vi "Configure Chan Input.vi"(6 "Gate Mode (0:Disabled)":T1(ring), 7 "Channel (1:Chan A)":i32(ring)=1 items=["Channel A"=1, "Channel B"=2, "Channel C"=3, "Channel D"=4, "Channel E"=5, "Channel F"=6, "Channel G"=7, "Channel H"=8], 8 "error in (no error)":errorcluster, 9 "Gate Logic (0:Disabled)":enum16{"Disabled", "Low", "High"}(ring), 10 "Sync Source (0:To)":i32(ring) items=["System (To)", "Channel A", "Channel B", "Channel C", "Channel D", "Channel E", "Channel F", "Channel G", "Channel H"], 11 "VISA resource name":refnum<visa-resource-name>) -> (0 "error out":errorcluster, 3 "VISA resource name out":refnum<visa-resource-name>)   [LabVIEW 2012, in "Berkeley Nucleonics 500 Series.lvlib"]
doc: "This VI is used to configure the gate mode for a channel."
uses:
  Berkeley Nucleonics 500 Series.lvlib
panel:
  # "The \"Gate Mode\" input is currently only utilized by 9520/9530 instruments.  When controlling a 9520/9530, the \"Gate Logic\" disabled setting is ignored."
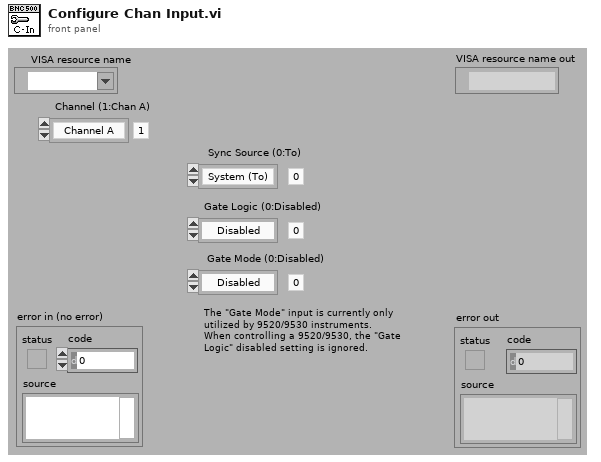
[diagram p1: front panel]
types:
  T1 = enum16{"Disabled", "Pulse Inhibit", "Output Inhibit"}
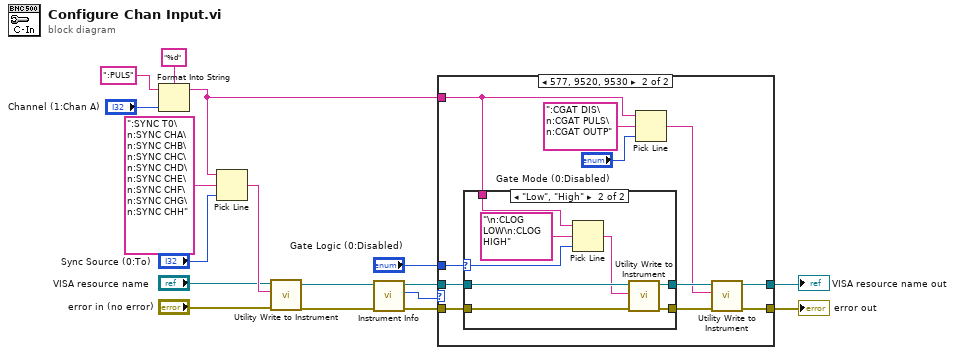
[diagram p0: block diagram]
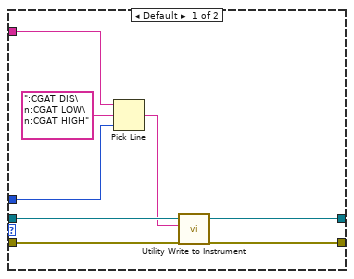
[diagram p2: hidden frame]
diagram:
  n1 = Format Into String(format string="%d", initial string=":PULS", "Channel (1:Chan A)") -> (resulting string=w5:string)  [unwired: 1 in, 1 out]
  n2 = Pick Line(string ("")=w5, multi-line string=":SYNC T0\n:SYNC CHA\n:SYNC CHB\n:SYNC CHC\n:SYNC CHD\n:SYNC CHE\n:SYNC CHF\n:SYNC CHG\n:SYNC CHH", line index="Sync Source (0:To)") -> (output string=w15:string)
  n3 = call "Utility Write to Instrument.vi"("error in (no error)"="error in (no error)", "Write Buffer"=w15, "VISA resource name"="VISA resource name") -> ("error out"=w11:errorcluster, "VISA resource name out"=w10:refnum<visa-resource-name>)  [unwired: 7 out]
  n4 = call "Instrument Info.vi"("error in (no error)"=w11, "VISA resource name"=w10) -> ("error out"=w3:errorcluster, "Instr Model"=w1:u32, "VISA resource name out"=w4:refnum<visa-resource-name>)  [unwired: 7 out]
  n5 = case shown="577, 9520, 9530" w1 {
    tunnel: [w25 w34] -> w9
    tunnel: [w23 w33] -> w8
    tunnel: w5 -> [w20 w27]
    tunnel: w4 -> [w22 w35]
    tunnel: w3 -> [w24 w36]
    tunnel: "Gate Logic (0:Disabled)" -> [w18 w28]
    frame Default {
      n6 = Pick Line(string ("")=w20, multi-line string=":CGAT DIS\n:CGAT LOW\n:CGAT HIGH", line index=w18) -> (output string=w19:string)
      n7 = call "Utility Write to Instrument.vi"("error in (no error)"=w24, "Write Buffer"=w19, "VISA resource name"=w22) -> ("error out"=w25:errorcluster, "VISA resource name out"=w23:refnum<visa-resource-name>)  [unwired: 7 out]
    }
    frame 577, 9520, 9530 {
      n8 = case shown="\"Low\", \"High\"" w28 {
        selector: w28 -> [_ w40]
        tunnel: [w37 w46] -> w31
        tunnel: w36 -> [w37 w43]
        tunnel: [w38 w45] -> w32
        tunnel: w35 -> [w38 w44]
        tunnel: w27 -> [_ w41]
        frame "Disabled" {
        }
        frame "Low", "High" {
          n9 = Pick Line(string ("")=w41, multi-line string="\n:CLOG LOW\n:CLOG HIGH", line index=w40) -> (output string=w39:string)
          n10 = call "Utility Write to Instrument.vi"("error in (no error)"=w43, "Write Buffer"=w39, "VISA resource name"=w44) -> ("error out"=w46:errorcluster, "VISA resource name out"=w45:refnum<visa-resource-name>)  [unwired: 7 out]
        }
      }
      n11 = Pick Line(string ("")=w27, multi-line string=":CGAT DIS\n:CGAT PULS\n:CGAT OUTP", line index="Gate Mode (0:Disabled)") -> (output string=w26:string)
      n12 = call "Utility Write to Instrument.vi"("error in (no error)"=w31, "Write Buffer"=w26, "VISA resource name"=w32) -> ("error out"=w34:errorcluster, "VISA resource name out"=w33:refnum<visa-resource-name>)  [unwired: 7 out]
    }
  }
  "error out" <- w9
  "VISA resource name out" <- w8
